vi "OpenURI - Basic Example.vi"() -> ()   [LabVIEW 2013]
uses:
  uri/URI.lvclass/URI.ctl
  components/path/URI-Component.Path.lvclass/URI-Component.Path.ctl
  components/path/URI-Component.Path.lvclass
  uri/Write scheme.vi
  uri/Write port.vi
  uri/Write host.vi
  uri/Read path.vi
  uri/Read path segments.vi
  components/path/Get Segments.vi
  uri/checkCached.vi
  components/path/Get path (absolute).vi
  uri/URI.lvclass
panel:
  out "port":u16
  out "Raw Segments":string[](array[string])
  out "Encoded Segments":string[](array[string])
  out "Raw Path":string
  out "Encoded Path":string
  out "set path with restricted characters":string
  out "set path by segments":string
  out "query from attributes":string
  out "changed scheme and port":string
  out "multiple query parameters":string
  out "query":string
  out "index.php":string
  out "Localhost URI":string
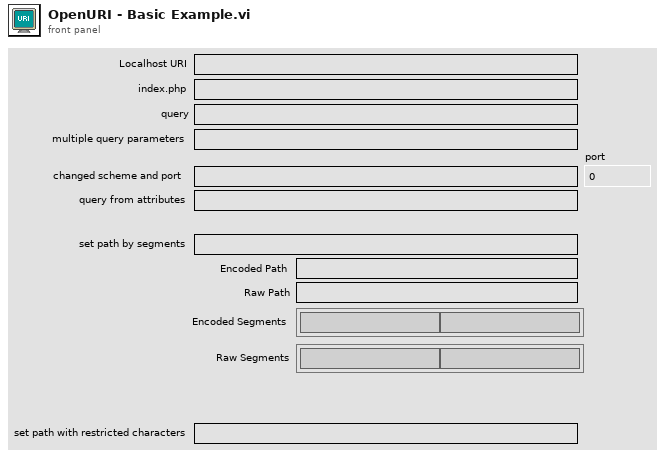
[diagram p1: front panel]
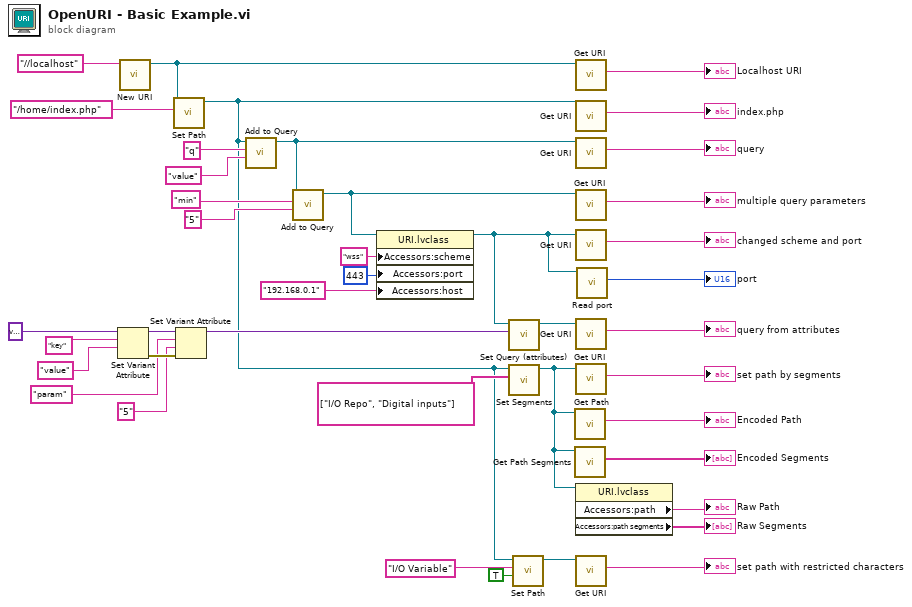
[diagram p0: block diagram]
diagram:
  n1 = Set Variant Attribute(Variant=variant ("variant"), name="key" ("path"), value="value" ("path")) -> (Variant out=w19:variant, error out=w20:errorcluster)  [unwired: 1 in, 1 out]
  n2 = call "New URI.vi"("URI"="//localhost") -> ("URI"=w39:refnum<class "URI.lvclass">)  [unwired: 9 in, 1 out]
  n3 = call "Set Path.vi"("path"="/home/index.php", "URI in"=w39) -> ("URI out"=w7:refnum<class "URI.lvclass">)  [unwired: 8 in, 1 out]
  n4 = Set Variant Attribute(Variant=w19, name="param" ("path"), value="5" ("path"), error in=w20) -> (Variant out=w16:variant)  [unwired: 2 out]
  n5 = call "Add to Query.vi"("value"="value" ("path"), "key"="q" ("path"), "URI in"=w7) -> ("URI out"=w33:refnum<class "URI.lvclass">)  [unwired: 7 in, 1 out]
  n6 = call "Add to Query.vi"("value"="5" ("path"), "key"="min" ("path"), "URI in"=w33) -> ("URI out"=w29:refnum<class "URI.lvclass">)  [unwired: 7 in, 1 out]
  n7 = property class="URI.lvclass"(reference=w29, "Accessors:scheme"="wss" ("scheme"), "Accessors:port"=u16 443 ("port"), "Accessors:host"="192.168.0.1" ("scheme")) -> (reference out=w3:refnum<class "URI.lvclass">)  [unwired: 1 in, 1 out]
  n8 = call "Set Query (attributes).vi"("Query"=w16, "URI in"=w3) -> ("URI out"=w24:refnum<class "URI.lvclass">)  [unwired: 8 in, 1 out]
  n9 = call "Set Segments.vi"("Segments"=string[] ["I/O Repo", "Digital inputs"], "URI in"=w7) -> ("URI out"=w6:refnum<class "URI.lvclass">)  [unwired: 8 in, 1 out]
  n10 = call "Set Path.vi"("Encode?"=TRUE, "path"="I/O Variable", "URI in"=w7) -> ("URI out"=w11:refnum<class "URI.lvclass">)  [unwired: 7 in, 1 out]
  n11 = call "Get Path.vi"("URI in"=w6) -> ("path"=→"Encoded Path":string)  [unwired: 8 in, 2 out]
  n12 = call "Get Path Segments.vi"("URI in"=w6) -> ("Segments"=→"Encoded Segments":string[])  [unwired: 8 in, 2 out]
  n13 = call "Get URI.vi"("URI in"=w39) -> ("URI String"=→"Localhost URI":string)  [unwired: 8 in, 2 out]
  n14 = call "Get URI.vi"("URI in"=w7) -> ("URI String"=→"index.php":string)  [unwired: 8 in, 2 out]
  n15 = call "Get URI.vi"("URI in"=w33) -> ("URI String"=→"query":string)  [unwired: 8 in, 2 out]
  n16 = call "Get URI.vi"("URI in"=w29) -> ("URI String"=→"multiple query parameters":string)  [unwired: 8 in, 2 out]
  n17 = call "Get URI.vi"("URI in"=w3) -> ("URI String"=→"changed scheme and port":string)  [unwired: 8 in, 2 out]
  n18 = call "Get URI.vi"("URI in"=w24) -> ("URI String"=→"query from attributes":string)  [unwired: 8 in, 2 out]
  n19 = call "Get URI.vi"("URI in"=w6) -> ("URI String"=→"set path by segments":string)  [unwired: 8 in, 2 out]
  n20 = property class="URI.lvclass"(reference=w6) -> ("Accessors:path"=→"Raw Path":string, "Accessors:path segments"=→"Raw Segments":string[])  [unwired: 1 in, 2 out]
  n21 = call "Get URI.vi"("URI in"=w11) -> ("URI String"=→"set path with restricted characters":string)  [unwired: 8 in, 2 out]
  n22 = call "Read port.vi"("URI in"=w3) -> ("port"=→"port":u16)  [unwired: 8 in, 2 out]
